vi "FlushQueue.vi"(3 "error in (no error)":errorcluster, 5 "nInputHandle":u64) -> (0 "error out":errorcluster, 1 "GX_STATUS":i32, 2 "nOutputHandle":u64)   [LabVIEW 2016, in "GxLVLib.lvlib"]
uses:
  GxLVLib.lvlib
  GxIAPI.dll
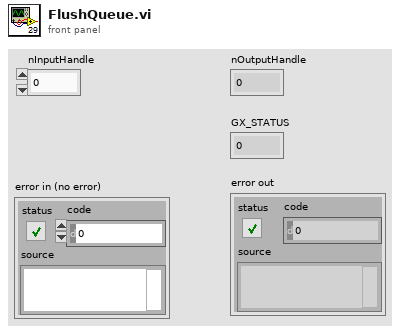
[diagram p1: front panel]
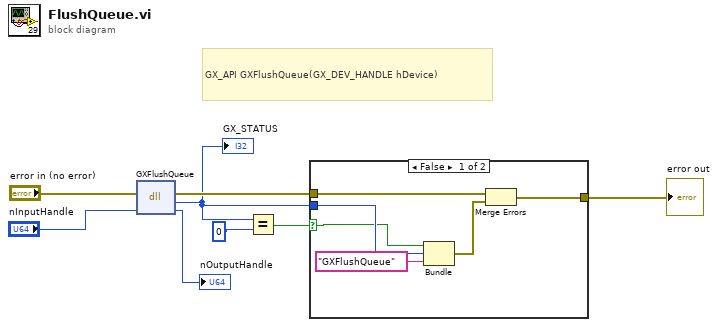
[diagram p0: block diagram]
diagram:
  # "GX_API GXFlushQueue(GX_DEV_HANDLE hDevice)"
  n1 = dll-call lib="GxIAPI.dll" fn="GXFlushQueue"(error in="error in (no error)", "hDevice"="nInputHandle") -> (error out=w4:errorcluster, "GX_STATUS"=w1:i32, "hDevice"=→"nOutputHandle":i64)  [unwired: 2 in, 1 out]
  "GX_STATUS" <- w1
  n2 = Equal?(x=w1, y=0) -> (x = y?=w3:bool)
  n3 = case shown="False" w3 {
    selector: w3 -> [w10 _]
    tunnel: w4 -> [w14 w15]
    tunnel: [w13 w15] -> w5
    tunnel: w1 -> [w11 _]
    frame False {
      n4 = Bundle(w10, "GX_STATUS"=w11, "GXFlushQueue") -> (w12:cluster{bool, "GX_STATUS":i32, string})  [unwired: 1 in]
      n5 = Merge Errors(w14, w12) -> (w13:errorcluster)
    }
    frame True {
    }
  }
  "error out" <- w5
